vi "ProcessOnDemandWaveform.vi"(7 "Qbus in":refnum<class "Qbus.lvclass">, 8 "error in (no error)":errorcluster, 10 "on demand waveform":T1, 11 "config in":T2={"DataSet Type"=enum."Waveform", "ChanNameMap"=variant, "Common"={"State"=enum."On", "Waveform Channel"="", "DataGroup"="", "Number of Samples"=0, "Waveform Length (sec)"=0.0, "Timeout"=0.0, "History"=variant, "LastRequest"=timestamp(0 s since 1904-01-01), "BufferSize"=0, "OpState"=variant, "IRoutingSource"={"CorrelationId"="", "ReplyTo"=""}}}) -> (0 "error out":errorcluster, 3 "config out":T2={"DataSet Type"=enum."Waveform", "ChanNameMap"=variant, "Common"={"State"=enum."On", "Waveform Channel"="", "DataGroup"="", "Number of Samples"=0, "Waveform Length (sec)"=0.0, "Timeout"=0.0, "History"=variant, "LastRequest"=timestamp(0 s since 1904-01-01), "BufferSize"=0, "OpState"=variant, "IRoutingSource"={"CorrelationId"="", "ReplyTo"=""}}})   [LabVIEW 2017, in "EmsaTestPanel.lvlib"]
uses:
  <vilib>/addons/InsightCM/Devices/Shared/Emsa/EmsaTestPanel/EmsaTestPanel.lvlib
  <vilib>/addons/InsightCM/Devices/Shared/Emsa/EmsaTestPanel/controls/Configuration.ctl
  <vilib>/addons/InsightCM/Devices/Shared/Emsa/EmsaTestPanel/controls/DataSetType.ctl
  <vilib>/addons/InsightCM/Devices/Shared/Common/TestPanel/controls/Configuration.ctl
  <vilib>/addons/InsightCM/Devices/Shared/Common/TestPanel/controls/State.ctl
  <vilib>/addons/InsightCM/MessageBus/Base/controls/IRoutingSource.ctl
  <vilib>/addons/Qbus/Qbus.lvclass
  <vilib>/addons/InsightCM/Devices/Shared/Emsa/EmsaAcquisition/controls/OnDemandWaveformData.ctl
  <vilib>/addons/InsightCM/MessageBus/MessageLibrary/Device/controls/DeviceTestPanelGetDataSetForChannelResponseBody.ctl
  <vilib>/addons/InsightCM/MessageBus/Base/controls/DataSetByteData.ctl
  <vilib>/addons/InsightCM/MessageBus/Base/controls/KeyValuePair.ctl
  <vilib>/addons/InsightCM/Devices/Shared/Common/ServerComm/ServerComm.lvlib
  <vilib>/addons/InsightCM/Devices/Shared/Common/TestPanel/TestPanel.lvlib
  <vilib>/addons/InsightCM/Devices/Shared/Emsa/EmsaAcquisition/EmsaAcquisition.lvlib
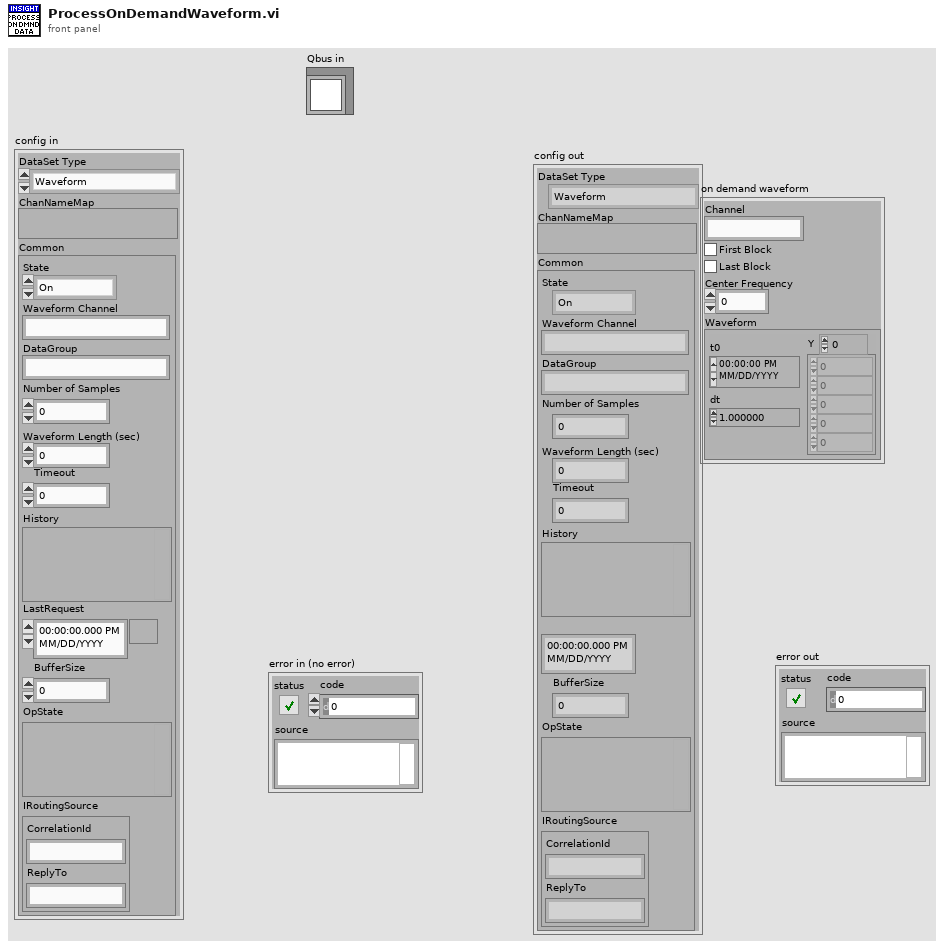
[diagram p1: front panel]
types:
  T1 = typedef "EmsaAcquisition.lvlib/OnDemandWaveformData.ctl" = cluster{"Channel":string, "First Block":bool, "Last Block":bool, "Center Frequency":dbl, "Waveform":waveform(dbl)}
  T2 = typedef "EmsaTestPanel.lvlib/Configuration.ctl" = cluster{"DataSet Type":T3, "ChanNameMap":variant, "Common":T4}
  T3 = typedef "EmsaTestPanel.lvlib/DataSetType.ctl" = enum16{"Waveform", "Sweep", "WAV"}
  T4 = typedef "TestPanel.lvlib/Configuration.ctl" = cluster{"State":T5, "Waveform Channel":string, "DataGroup":string, "Number of Samples":i32, "Waveform Length (sec)":dbl, "Timeout":dbl, "History":variant, "LastRequest":timestamp, "BufferSize":i32, "OpState":variant, "IRoutingSource":T6}
  T5 = typedef "TestPanel.lvlib/State.ctl" = enum16{"Off", "On", "PendingValues", "PendingDataSet"}
  T6 = typedef "IRoutingSource.ctl" = cluster{"CorrelationId":string, "ReplyTo":string}
  T7 = typedef "DeviceTestPanelGetDataSetForChannelResponseBody.ctl" = cluster{"DataSet":T8}
  T8 = typedef "DataSetByteData.ctl" = cluster{"Id":string, "DataEventId":string, "AssetNodeId":string, "Type":string, "T0":i64, "Props":T9[], "DataBase64":string}
  T9 = typedef "KeyValuePair.ctl" = cluster{"Key":string, "Value":string}
  T10 = typedef "Message.ctl" = cluster{"Header":T11, "Body":u8[]}
  T11 = typedef "MessageHeader.ctl" = cluster{"MessageName":string, "Timestamp":i64, "CorrelationId":string, "ContentType":string, "RoutingKey":string, "Properties":T9[]}
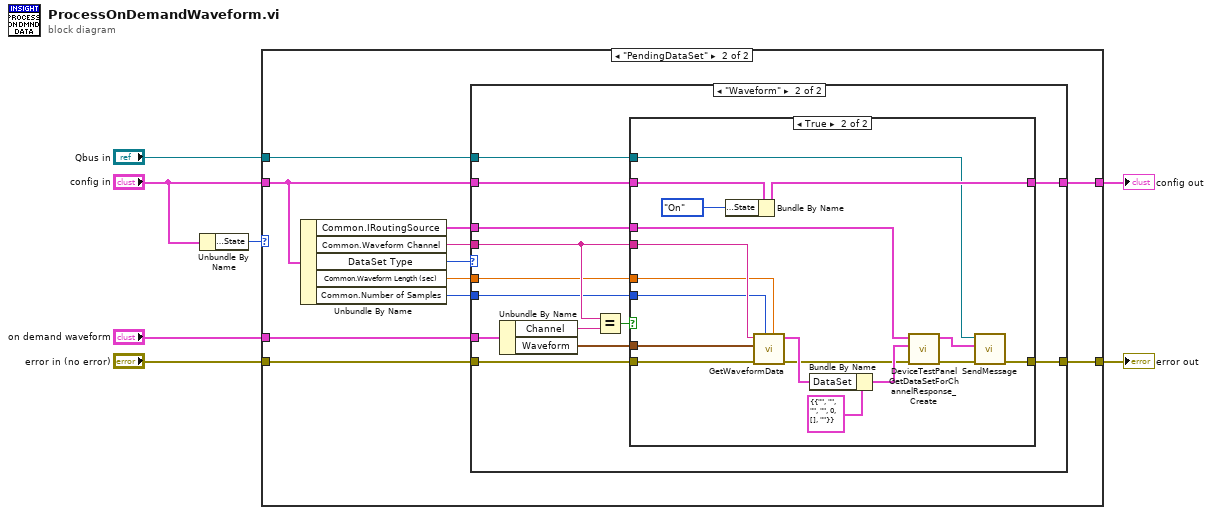
[diagram p0: block diagram]
diagram:
  n1 = Unbundle By Name("config in") -> ("Common.State"=w7:T5)
  n2 = case shown="\"PendingDataSet\"" w7 {
    tunnel: "error in (no error)" -> [w8 w20]
    tunnel: [w8 w15] -> w3
    tunnel: "config in" -> [w9 w18]
    tunnel: [w9 w17] -> w4
    tunnel: "Qbus in" -> [_ w16]
    tunnel: "on demand waveform" -> [_ w12]
    frame Default {
    }
    frame "PendingDataSet" {
      n3 = Unbundle By Name(w18) -> ("Common.IRoutingSource"=w14:T6, "Common.Waveform Channel"=w19:string, "DataSet Type"=w13:T3, "Common.Waveform Length (sec)"=w11:dbl, "Common.Number of Samples"=w10:i32)
      n4 = case shown="\"Waveform\"" w13 {
        tunnel: w20 -> [w21 w35]
        tunnel: w19 -> [_ w27]
        tunnel: w18 -> [w22 w34]
        tunnel: [w22 w33] -> w17
        tunnel: w16 -> [_ w32]
        tunnel: [w21 w31] -> w15
        tunnel: w14 -> [_ w30]
        tunnel: w12 -> [_ w29]
        tunnel: w11 -> [_ w23]
        tunnel: w10 -> [_ w24]
        frame Default {
        }
        frame "Waveform" {
          n5 = Unbundle By Name(w29) -> ("Channel"=w28:string, "Waveform"=w25:waveform(dbl))
          n6 = Equal?(x=w27, y=w28) -> (x = y?=w26:bool)
          n7 = case shown="True" w26 {
            tunnel: w35 -> [w37 w43]
            tunnel: w27 -> [_ w40]
            tunnel: w34 -> [w36 w54]
            tunnel: [w36 w53] -> w33
            tunnel: w32 -> [_ w52]
            tunnel: [w37 w49] -> w31
            tunnel: w30 -> [_ w47]
            tunnel: w25 -> [_ w41]
            tunnel: w24 -> [_ w39]
            tunnel: w23 -> [_ w38]
            frame False {
            }
            frame True {
              n8 = Bundle By Name(cluster=w54, "Common.State"=State."On" ("Test Panel State")) -> (w53:T2)
              n9 = call <vilib>:"GetWaveformData.vi"("Waveform Length (sec)"=w38, "Number of Samples"=w39, "error in (no error)"=w43, "Waveform"=w41, "Channel"=w40) -> ("error out"=w42:errorcluster, "DataSet"=w44:T8)  [unwired: 5 in]
              n10 = Bundle By Name(cluster=T7 {"DataSet"={"Id"="", "DataEventId"="", "AssetNodeId"="", "Type"="", "T0"=0, "Props"=[], "DataBase64"=""}} ("DeviceTestPanelGetWaveformChannelResponse"), "DataSet"=w44) -> (w48:T7)
              n11 = call <vilib>:"DeviceTestPanelGetDataSetForChannelResponse_Create.vi"("error in (no error)"=w42, "DeviceTestPanelGetDataSetForChannelResponse"=w48, "IRoutingSource"=w47) -> ("error out"=w50:errorcluster, "Message"=w46:T10)  [unwired: 7 in]
              n12 = call <vilib>:"SendMessage.vi"("error in (no error)"=w50, "message"=w46, "Qbus in"=w52) -> ("error out"=w49:errorcluster)  [unwired: 7 in, 1 out]
            }
          }
        }
      }
    }
  }
  "error out" <- w3
  "config out" <- w4
